vi "rpm_using_escon.vi"(11 "AI":dbl[](array[slide]) scale=-4.0..4.0) -> (3 "rpm":i32[](array[knob]) scale=0.0..10.0)   [LabVIEW 2021]
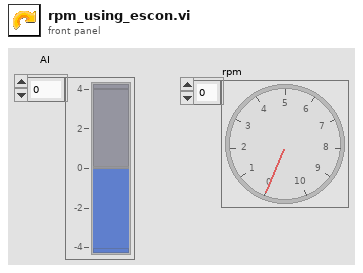
[diagram p1: front panel]
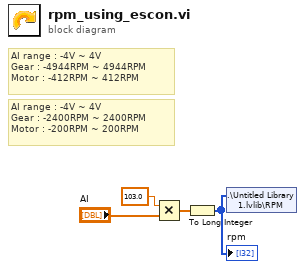
[diagram p0: block diagram]
diagram:
  # "AI range : -4V ~ 4V\nGear : -4944RPM ~ 4944RPM\nMotor : -412RPM ~ 412RPM"
  # "AI range : -4V ~ 4V\nGear : -2400RPM ~ 2400RPM\nMotor : -200RPM ~ 200RPM"
  n1 = Multiply(x=103.0, y="AI") -> (x*y=w2:dbl[])
  n2 = To Long Integer(number=w2) -> (32bit integer=w1:i32[])
  "rpm" <- w1
  n3 = shared-variable ".\\Untitled Library 1.lvlib\\RPM"(w1) -> ()  [unwired: 1 in, 1 out]
